vi "Get Unique Name.vi"(8 "error in (no error)":errorcluster, 11 "Object Layout in":refnum<class "Object Layout.lvclass">) -> (0 "error out":errorcluster, 1 "found?":bool, 2 "unique name":string, 3 "Object Layout out":refnum<class "Object Layout.lvclass">)   [LabVIEW 2010, in "NI_SE_Front Panel Layout.lvlib" / "Object Layout.lvclass"]
uses:
  Object Layout.lvclass
  Object Layout.lvclass/Object Layout.ctl
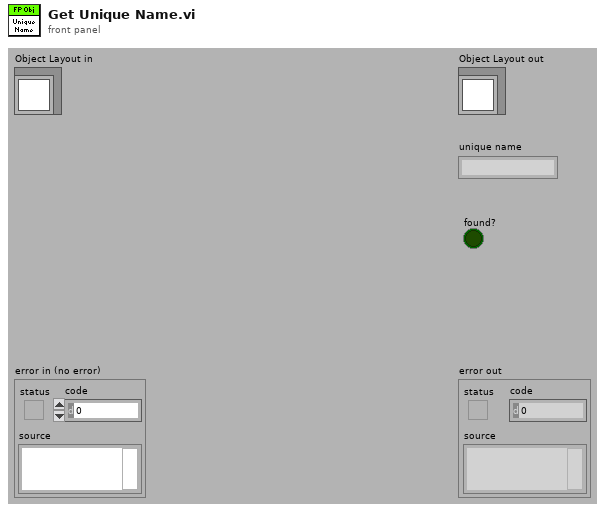
[diagram p1: front panel]
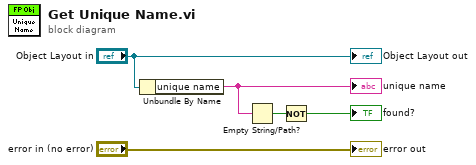
[diagram p0: block diagram]
diagram:
  n1 = Unbundle By Name("Object Layout in") -> ("unique name"=w3:string)
  "unique name" <- w3
  n2 = Empty String/Path?(string/path=w3) -> (empty?=w2:bool)
  n3 = Not(x=w2) -> (.not. x?=→"found?":bool)
  "error out" <- "error in (no error)"
  "Object Layout out" <- "Object Layout in"
